vi "getConnectionPoint.vi"(0 "reference":refnum<class "ImplicitParameterNode.lvclass">, 1 "direction":refnum<class "Direction.lvclass">, 5 "error in (no error)":errorcluster) -> (14 "reference out":refnum<class "ImplicitParameterNode.lvclass">, 15 "point2D":T1 {"y" format="%.2f"; "x" format="%.2f"}, 19 "error out":errorcluster)   [LabVIEW 2012, in "ImplicitParameterNode.lvclass"]
doc: "public Point2D getConnectionPoint(Direction d)"
uses:
  <resource>/Framework/Providers/Open_GDS/UML/ImplicitParameterNode_class/ImplicitParameterNode.lvclass
  <resource>/Framework/Providers/Open_GDS/UML/Direction_class/Direction.lvclass
  <resource>/Framework/Providers/Open_GDS/UML/General/Point/Point Point2D.ctl
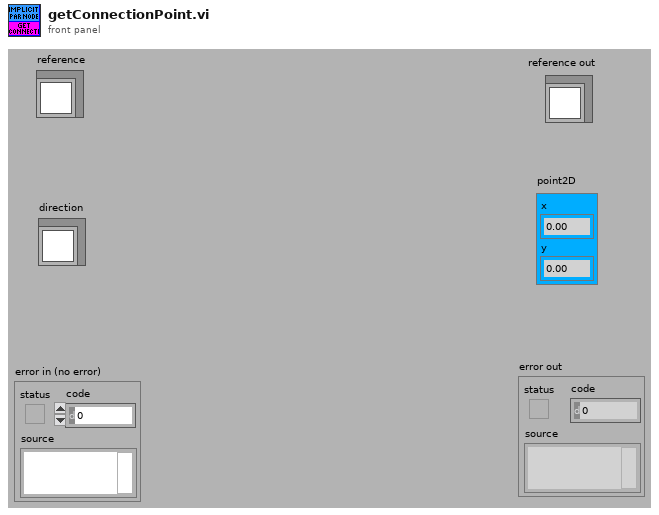
[diagram p1: front panel]
types:
  T1 = typedef "Point Point2D.ctl" = cluster{"x":dbl, "y":dbl}
  T2 = typedef "ImplicitParameterNode.lvclass/ObjectAttributes.ctl" = cluster{"Base class":T3, "topHeight":dbl, "name":refnum<class "MultiLineString.lvclass">, "DEFAULT_TOP_HEIGHT":i32, "DEFAULT_WIDTH":i32, "DEFAULT_HEIGHT":i32}
  T3 = typedef "RectangularNode.lvclass/ObjectAttributes.ctl" = cluster{"Base class":T4, "bounds":T5}
  T4 = typedef "AbstractNode.lvclass/ObjectAttributes.ctl" = cluster{"parent":refnum<class "AbstractNode.lvclass">, "children":refnum<class "AbstractNode.lvclass">[], "Hidden":bool}
  T5 = typedef "Rectangle Rectangle2D.ctl" = cluster{"x":dbl, "y":dbl, "width":dbl, "height":dbl}
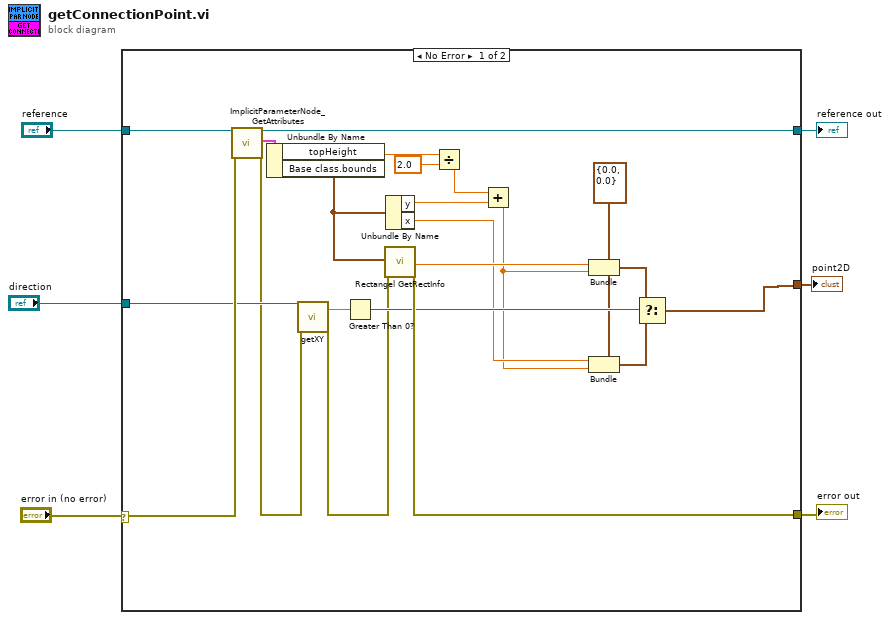
[diagram p0: block diagram]
diagram:
  n1 = case shown="No Error" "error in (no error)" {
    selector: "error in (no error)" -> [w25 w29]
    tunnel: "reference" -> [w28 w30]
    tunnel: [w27 w29] -> w5
    tunnel: [w26 w30] -> w4
    tunnel: [w24 _] -> w2
    tunnel: "direction" -> [w23 _]
    frame No Error {
      w18 = T1 {"x"=0.0, "y"=0.0} ("point2D")
      n2 = call <resource>:"ImplicitParameterNode_GetAttributes.vi"("reference in"=w28, "error in (no error)"=w25) -> ("reference out"=w26:refnum<class "ImplicitParameterNode.lvclass">, "Attributes"=w22:T2, "error out"=w20:errorcluster)  [unwired: 15 out]
      n3 = Unbundle By Name(w22) -> ("topHeight"=w13:dbl, "Base class.bounds"=w15:T5)
      n4 = call <resource>:"getXY.vi"("reference"=w23, "error in (no error)"=w20) -> ("x"=w21:dbl, "error out"=w7:errorcluster)  [unwired: 16 out]
      n5 = Greater Than 0?(x=w21) -> (x > 0?=w19:bool)
      n6 = call <resource>:"Rectangel GetRectInfo.vi"("bounds"=w15, "error in (no error)"=w7) -> ("maxX"=w16:dbl, "error out"=w27:errorcluster)  [unwired: 16 out]
      n7 = Unbundle By Name(w15) -> ("y"=w14:dbl, "x"=w9:dbl)
      n8 = Divide(x=w13, y=2.0) -> (x/y=w11:dbl)
      n9 = Add(x=w11, y=w14) -> (x+y=w8:dbl)
      n10 = Bundle(cluster=w18, "x"=w16, "y"=w8) -> (w17:T1)
      n11 = Bundle(cluster=w18, "x"=w9, "y"=w8) -> (w10:T1)
      n12 = Select(t=w17, s=w19, f=w10) -> (s? t:f=w24:T1)
    }
    frame Error {
    }
  }
  "reference out" <- w4
  "error out" <- w5
  "point2D" <- w2
